vi "Set current pretomo stack.vi"(6 "z step number":i32, 8 "error in (no error)":errorcluster, 9 "current y stack":i32, 10 "current x stack":i32, 11 "Tomo in":refnum<class "Tomo.lvclass">) -> (0 "error out":errorcluster, 3 "Tomo out":refnum<class "Tomo.lvclass">)   [LabVIEW 2012, in "Tomo.lvclass"]
uses:
  Tomo.lvclass
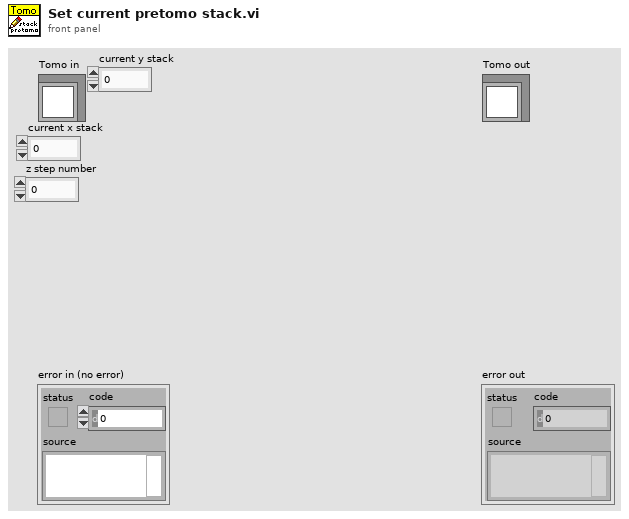
[diagram p1: front panel]
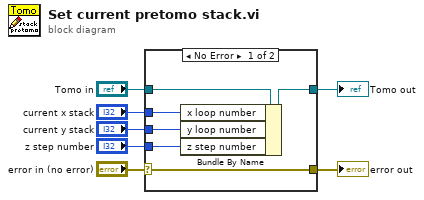
[diagram p0: block diagram]
diagram:
  n1 = case shown="No Error" "error in (no error)" {
    selector: "error in (no error)" -> [w13 w15]
    tunnel: [w13 w15] -> w6
    tunnel: [w11 w14] -> w4
    tunnel: "Tomo in" -> [w12 w14]
    tunnel: "current x stack" -> [w10 _]
    tunnel: "current y stack" -> [w9 _]
    tunnel: "z step number" -> [w8 _]
    frame No Error {
      n2 = Bundle By Name(cluster=w12, "x loop number"=w10, "y loop number"=w9, "z step number"=w8) -> (w11:refnum<class "Tomo.lvclass">)
    }
    frame Error {
    }
  }
  "error out" <- w6
  "Tomo out" <- w4
